vi "test.vi"   [LabVIEW 2023]
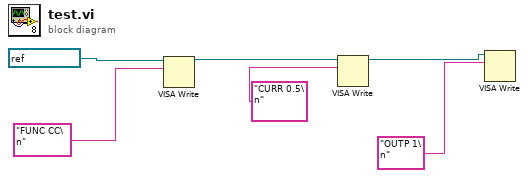
[diagram p0: block diagram]
diagram:
  n1 = VISA Write(VISA resource name=refnum<visa-resource-name> "FT6301A", write buffer="FUNC CC\n") -> (VISA resource name out=w4:refnum<visa-resource-name>)  [unwired: 1 in, 2 out]
  n2 = VISA Write(VISA resource name=w4, write buffer="CURR 0.5\n") -> (VISA resource name out=w2:refnum<visa-resource-name>)  [unwired: 1 in, 2 out]
  n3 = VISA Write(VISA resource name=w2, write buffer="OUTP 1\n") -> ()  [unwired: 1 in, 3 out]
